vi "DSF.Engine.Memory.Pointer.Array.Get Element Count.vi"(8 "error in (no error)":errorcluster, 11 "Array Pointer in":refnum<class "DSF.Engine.Memory.Pointer.Array.lvclass">) -> (0 "error out":errorcluster, 2 "element count":u64 format="%d elements", 3 "Array Pointer out":refnum<class "DSF.Engine.Memory.Pointer.Array.lvclass">)   [LabVIEW 2016, in "DSF.Engine.lvlib" / "DSF.Engine.Memory.Pointer.Array.lvclass"]
uses:
  Memory.Pointer/DSF.Engine.Memory.Pointer.Array.lvclass
  Memory.Pointer/DSF.Engine.Memory.Pointer.Array.lvclass/DSF.Engine.Memory.Pointer.Array.ctl
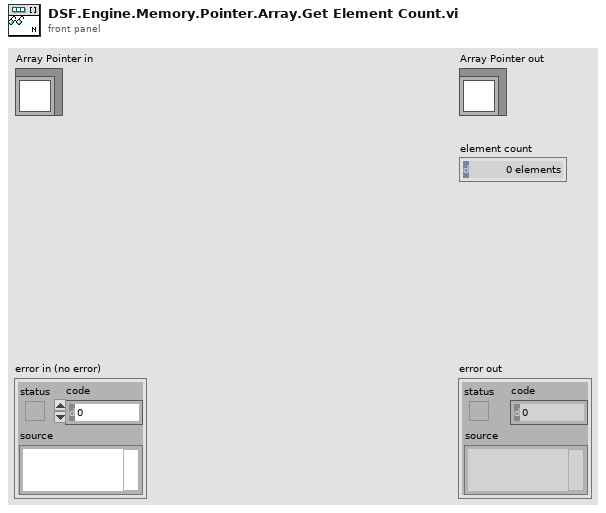
[diagram p1: front panel]
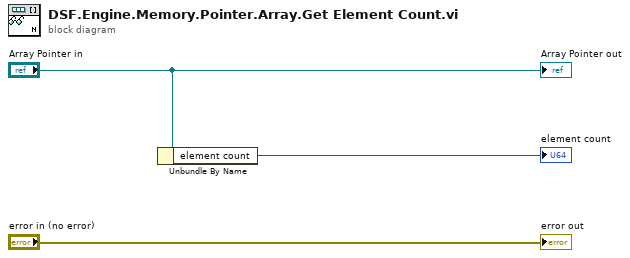
[diagram p0: block diagram]
diagram:
  n1 = Unbundle By Name("Array Pointer in") -> ("element count"=→"element count":u64)
  "error out" <- "error in (no error)"
  "Array Pointer out" <- "Array Pointer in"
